vi "The Grid.vi"(11 "Grid in":refnum<class "Grid.lvclass">) -> (3 "Grid.lvclass":refnum<class "Grid.lvclass">)   [LabVIEW 2016]
uses:
  Classes/Grid/Grid.lvclass
panel:
  out "Control Loop Count":i32
  out "Iteration Loop Count":i32
  in  "stop 2":bool
  in  "stop":bool
  in  "State":enum16{"Exit", "Generate Image"}(ring)
  in  "Color Array":u32[](array[colorbox])=[16711680, 16448250, 16860]
  in  "Grid Properties":T1={"Width"=400, "Height"=600, "Top Left Coordinate"=-1.4+0.2i, "Bottom Right Coordinate"=-1.2+0.22i}
  in  "input cluster 4":T1={"Width"=320, "Height"=240, "Top Left Coordinate"=1.0-2.5i, "Bottom Right Coordinate"=-1.0+1.0i}
  in  "input cluster 3":T1={"Width"=320, "Height"=240, "Top Left Coordinate"=1.0-2.5i, "Bottom Right Coordinate"=-1.0+1.0i}
  in  "input cluster 2":T1={"Width"=320, "Height"=240, "Top Left Coordinate"=-1.4+0.2i, "Bottom Right Coordinate"=-1.0+0.22i}
  out "new picture":picture
  in  "input cluster":T1={"Width"=320, "Height"=240, "Top Left Coordinate"=-1.112+0.21i, "Bottom Right Coordinate"=-1.104+0.25i}
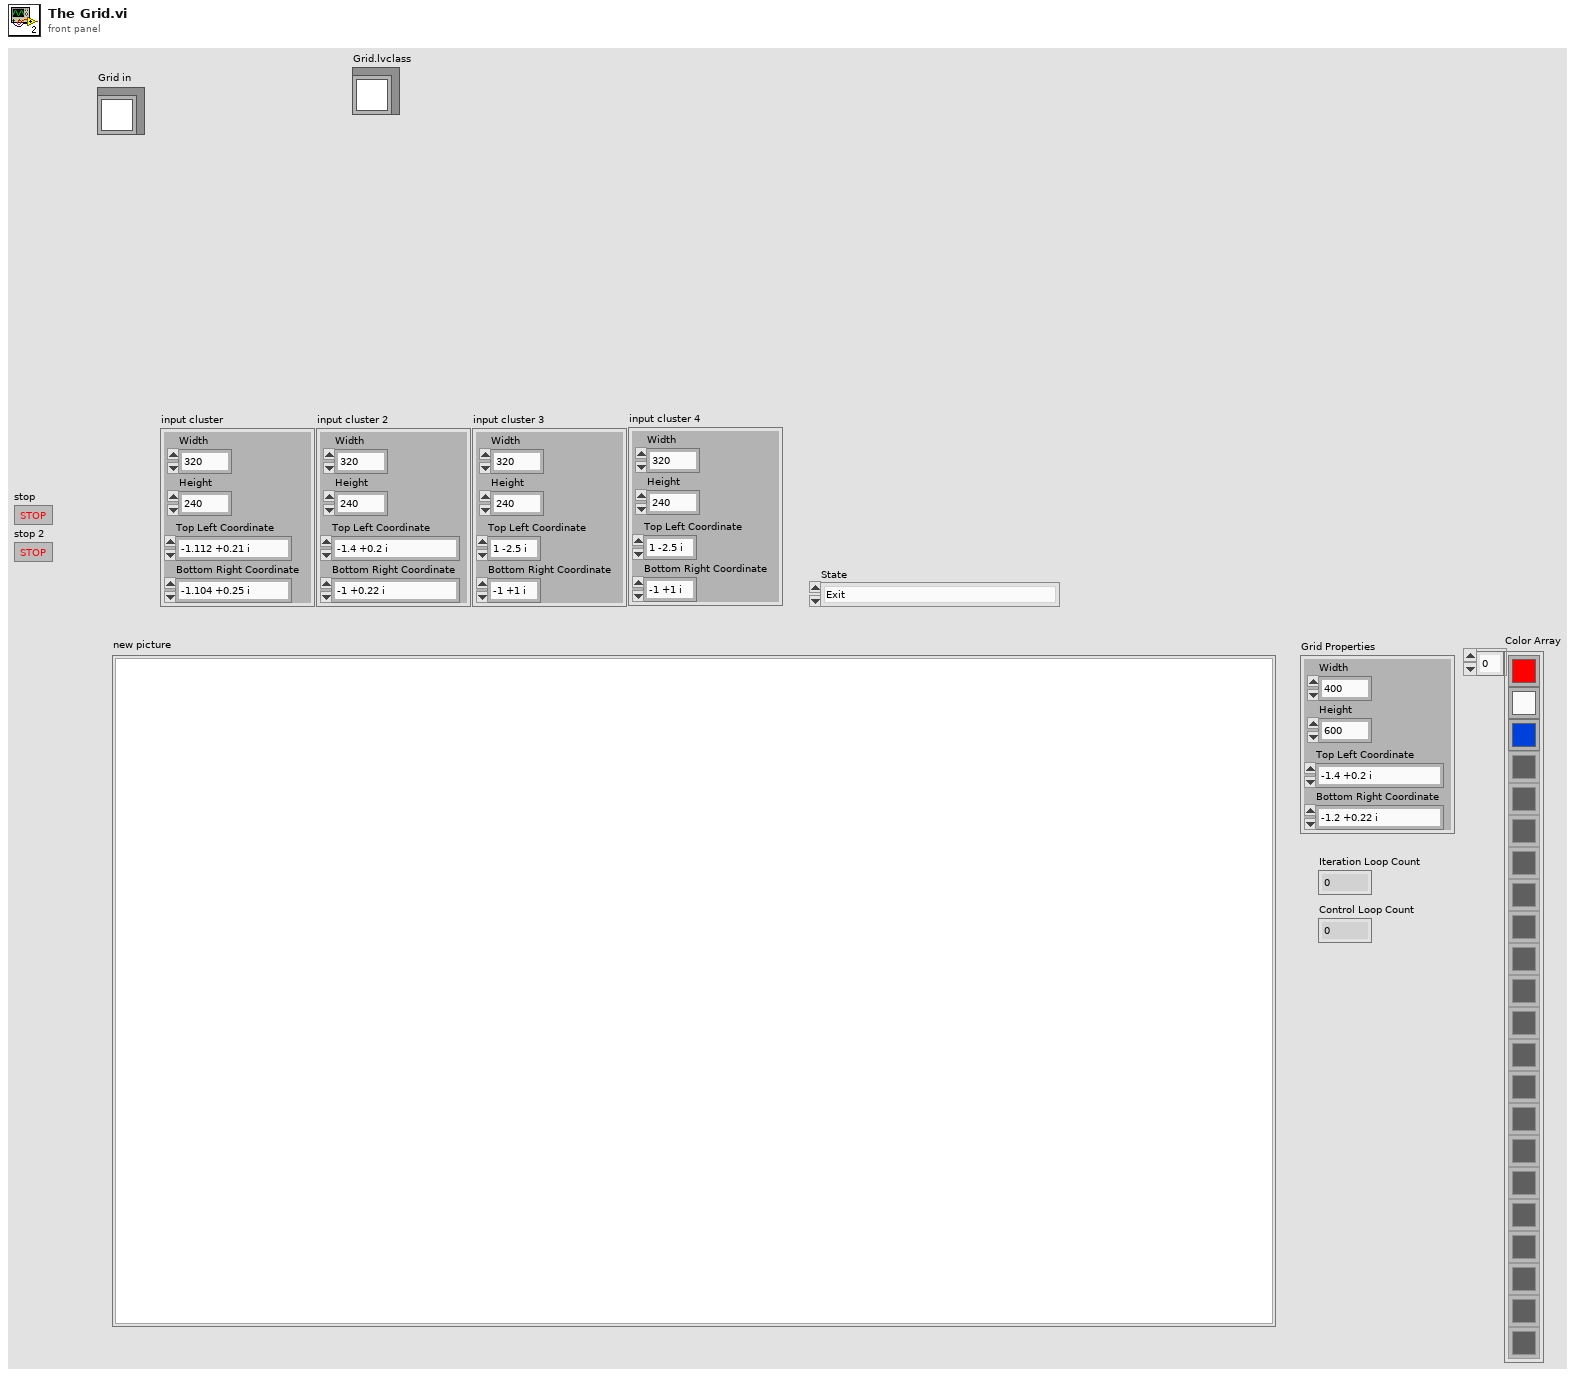
[diagram p1: front panel]
types:
  T1 = cluster{"Width":i32, "Height":i32, "Top Left Coordinate":cdb, "Bottom Right Coordinate":cdb}
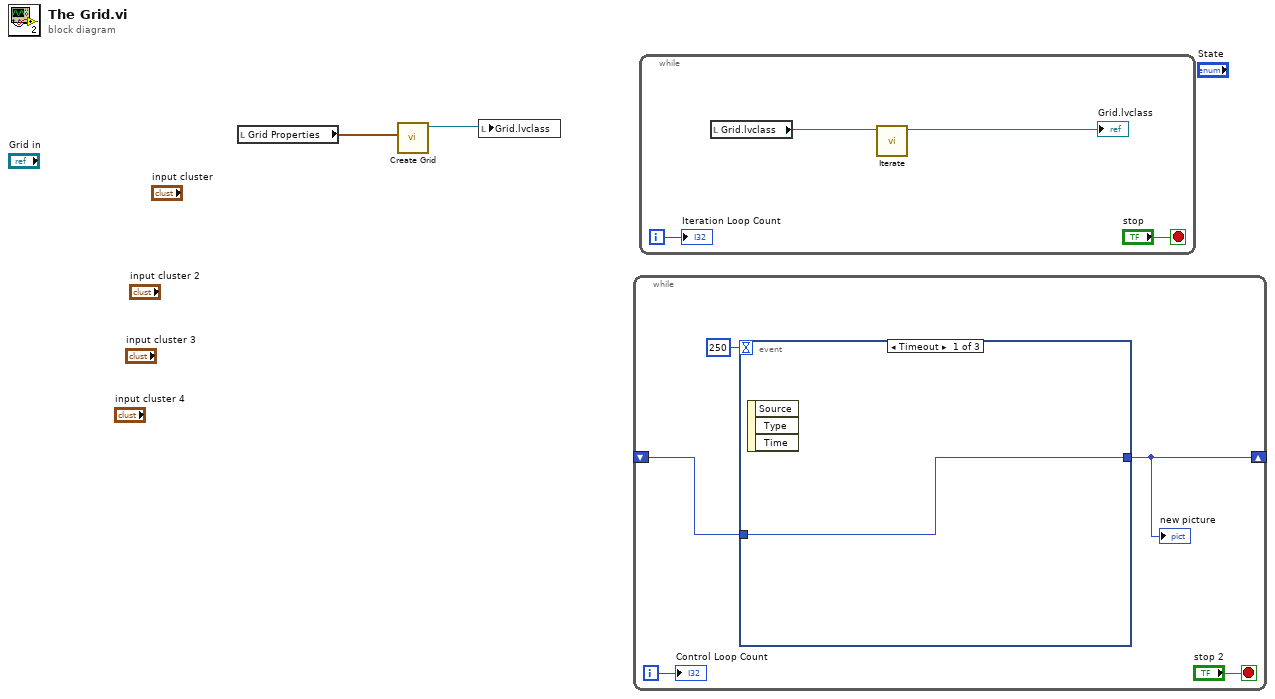
[diagram p0: block diagram]
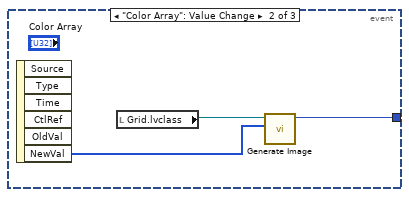
[diagram p2: hidden frame]
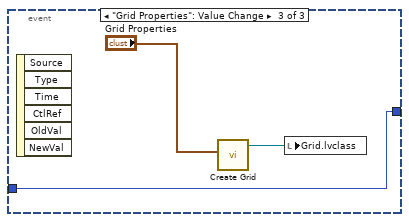
[diagram p3: hidden frame]
diagram:
  n1 = local read "Grid Properties"() -> (w2:T1)
  n2 = call "Create Grid.vi"("input cluster"=w2) -> ("Grid out"=w1:refnum<class "Grid.lvclass">)  [unwired: 10 in]
  n3 = local write "Grid.lvclass"(w1) -> ()
  n4 = while {
    shift-right: [w7] -> _
    shift-left: _ -> [w6]
    i -> [w3]
    stop <- "stop 2" stop-if-true
    n5 = event shown="[0] Timeout" {
      selector: _ -> [_ _ _]
      dyn-events: _ -> [_ _ _]
      timeout: 250 -> [_ _ _]
      tunnel: [w8 w9 w12] -> w7
      tunnel: w6 -> [w8 _ w12]
      event Timeout {
        n6 = event-data() -> ()  [unwired: 1 in, 3 out]
      }
      event "Color Array": Value Change {
        n7 = event-data() -> ("NewVal"=w10:u32[])  [unwired: 1 in, 5 out]
        n8 = local read "Grid.lvclass"() -> (w11:refnum<class "Grid.lvclass">)
        n9 = call "Generate Image.vi"("Color Array"=w10, "Grid.lvclass"=w11) -> ("new picture"=w9:picture)  [unwired: 9 in]
      }
      event "Grid Properties": Value Change {
        n10 = event-data() -> ()  [unwired: 1 in, 6 out]
        n11 = call "Create Grid.vi"("input cluster"="Grid Properties") -> ("Grid out"=w13:refnum<class "Grid.lvclass">)  [unwired: 10 in]
        n12 = local write "Grid.lvclass"(w13) -> ()
      }
    }
    "new picture" <- w7
    "Control Loop Count" <- w3
  }
  n13 = while {
    i -> [w15]
    stop <- "stop" stop-if-true
    n14 = local read "Grid.lvclass"() -> (w17:refnum<class "Grid.lvclass">)
    n15 = call "Iterate.vi"("Grid.lvclass 2"=w17) -> ("Grid.lvclass"=→"Grid.lvclass":refnum<class "Grid.lvclass">)  [unwired: 10 in]
    "Iteration Loop Count" <- w15
  }
